vi "RegisterVIs.vi"(8 "error in":errorcluster, 10 "VI References":refnum<vi>[](array[refnum])) -> (0 "error out":errorcluster, 1 "Current Language":string)   [LabVIEW 2017, in "JKI Simple Localization.lvlib"]
doc: "Register VI(s) to the localizer's registry. Automatically applies the current language to these VIs."
uses:
  API/JKI Simple Localization.lvlib
  Definitions/Private/Translation.Action.ctl
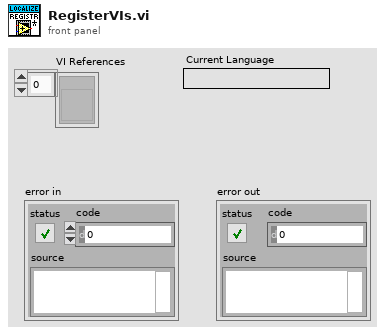
[diagram p1: front panel]
types:
  T1 = typedef "JKI Simple Localization.lvlib/Translation.Action.ctl" = enum16{"Read Dictionary", "Translate VIs", "Register VI", "Get Languages", "Translate Phrase", "Translate VI", "Unregister"}
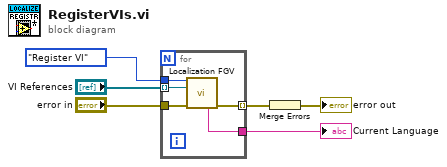
[diagram p0: block diagram]
diagram:
  n1 = for {
    tunnel: Translation.Action."Register VI" ("Action") -> [w11]
    tunnel: "error in" -> [w10]
    tunnel: [w9] -> w4 mode=indexing
    tunnel: "VI References" -> [w8] mode=indexing
    tunnel: [w7] -> w1
    n2 = call "Localization FGV.vi"("Action"=w11, "VI in"=w8, "error in"=w10) -> ("Current Language"=w7:string, "error out"=w9:errorcluster)  [unwired: 8 in, 3 out]
  }
  "Current Language" <- w1
  n3 = Merge Errors(w4) -> (→"error out":errorcluster)
